vi "MatFIle - Get.vi"(4 "error in":errorcluster) -> (0 "error out":errorcluster, 1 "NaN/Path/Refnum?":bool, 3 "storage refnum (file) out":refnum<k20>)   [LabVIEW 2023]
uses:
  controls/Action Enum.ctl
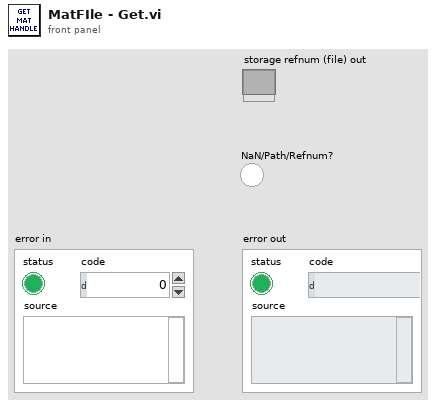
[diagram p1: front panel]
types:
  T1 = typedef "Action Enum.ctl" = enum16{"GET", "SET", "RESET"}
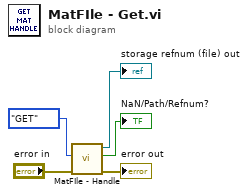
[diagram p0: block diagram]
diagram:
  n1 = call "MatFIle - Handle.vi"("error in"="error in", "Action Enum"=Action_Enum."GET") -> ("error out"=→"error out":errorcluster, "NaN/Path/Refnum?"=→"NaN/Path/Refnum?":bool, "storage refnum (file) out"=→"storage refnum (file) out":refnum<k20>)  [unwired: 3 in]
